vi "Page1.vi"(7 "LabVIEW Web Service Request":refnum<class "Web Request.lvclass">) -> ()   [LabVIEW 2020]
uses:
  <vilib>/wsapi/Web Request.lvclass
panel:
  # "Use the Web Service Request input terminal to call the VIs on the Web Services palette. Do not remove it from the connector pane unless you don't need access to the palette."
  # "Each additional control wired to the connector pane will be available as an input in the URL. To include an indicator in terminal-mode output (the default setting), it must also be wired to the connector pane."
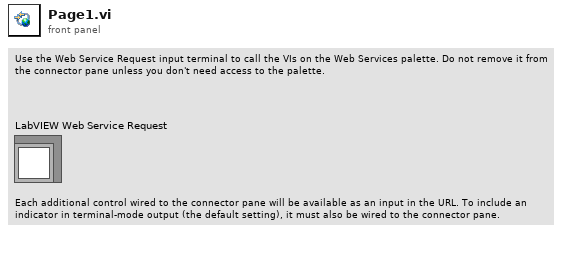
[diagram p1: front panel]
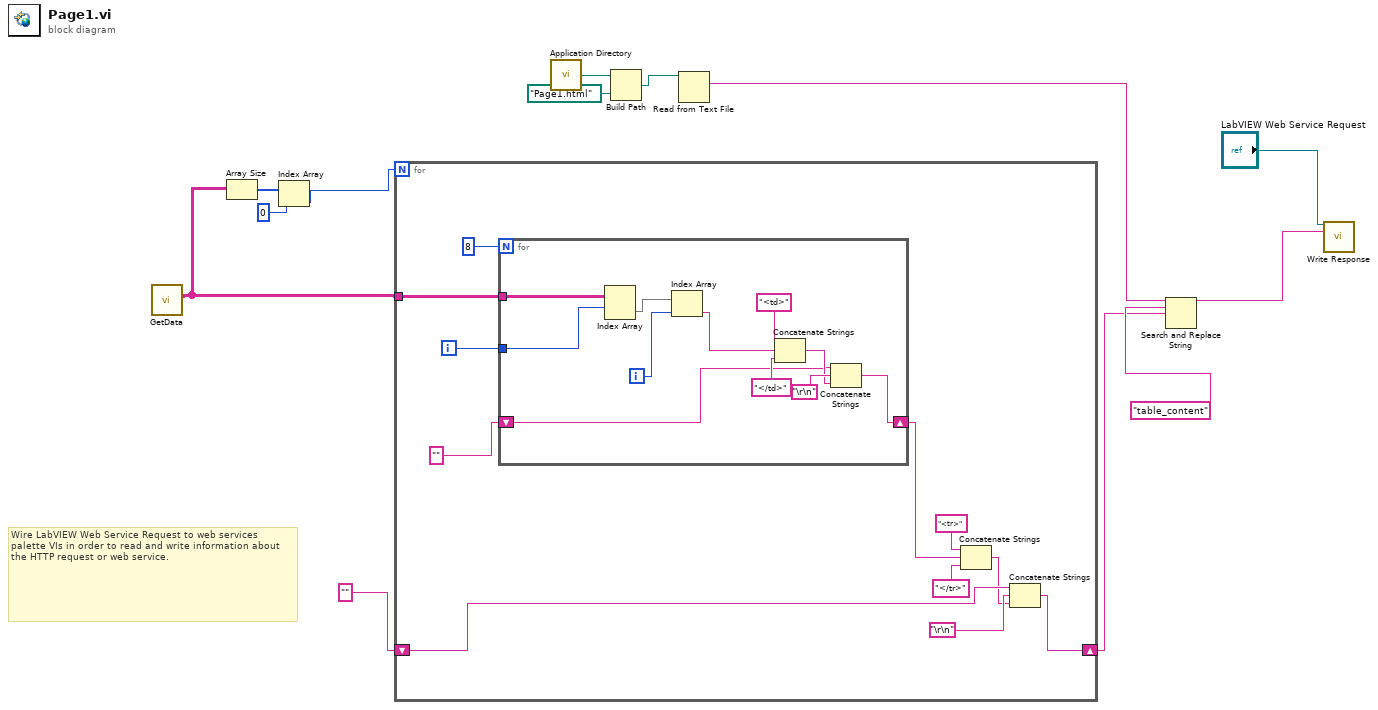
[diagram p0: block diagram]
diagram:
  # "Wire LabVIEW Web Service Request to web services palette VIs in order to read and write information about the HTTP request or web service."
  n1 = call "GetData.vi"() -> ("data"=w1:string[][])  [unwired: 11 in]
  n2 = Array Size(array=w1) -> (size(s)=w3:i32[])
  n3 = Index Array(array=w3, index=0) -> (element=w2:i32)
  n4 = for {
    N: w2 -> [_]
    shift-right: [w18] -> w5
    shift-left: "" ("search string") -> [w16]
    tunnel: w1 -> [w14]
    i -> [w22]
    n5 = for {
      N: 8 -> [_]
      shift-right: [w30] -> w19
      shift-left: "" ("search string") -> [w26]
      tunnel: w22 -> [w28]
      tunnel: w14 -> [w25]
      i -> [w35]
      n6 = Index Array(array=w25, index (row)=w28) -> (element=w34:string[])  [unwired: 1 in]
      n7 = Index Array(array=w34, index=w35) -> (element=w33:string)
      n8 = Concatenate Strings("<td>" ("search string"), w33, "</td>" ("search string")) -> (w27:string)
      n9 = Concatenate Strings(w26, "\r\n", w27) -> (w30:string)
    }
    n10 = Concatenate Strings("<tr>" ("search string"), w19, "</tr>" ("search string")) -> (w15:string)
    n11 = Concatenate Strings(w16, "\r\n", w15) -> (w18:string)
  }
  n12 = call <vilib>:"Application Directory.vi"() -> ("Application Directory"=w13:path)
  n13 = Build Path(base path=w13, name or relative path=path "Page1.html") -> (appended path=w11:path)
  n14 = Read from Text File(file (use dialog)=w11) -> (text=w7:string)  [unwired: 3 in, 3 out]
  n15 = Search and Replace String(input string=w7, search string="table_content", replace string=w5) -> (result string=w10:string)  [unwired: 5 in, 3 out]
  n16 = call <vilib>:"Write Response.vi"("LabVIEW Web Service Request"="LabVIEW Web Service Request", "response string"=w10) -> ()  [unwired: 12 in, 2 out]
